vi "Read String.vi"(8 "error in (no error)":errorcluster, 9 "offset (0)":i64, 10 "bytes to read":i64, 11 "pointer in":u64) -> (0 "error out":errorcluster, 1 "offset out":i64, 2 "string out":string, 3 "pointer out":u64)   [LabVIEW 2013, in "Linux RT IPC.Shared Memory.lvlib"]
uses:
  Linux RT IPC.Shared Memory.lvlib
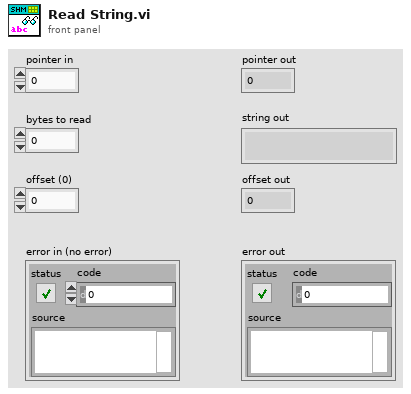
[diagram p1: front panel]
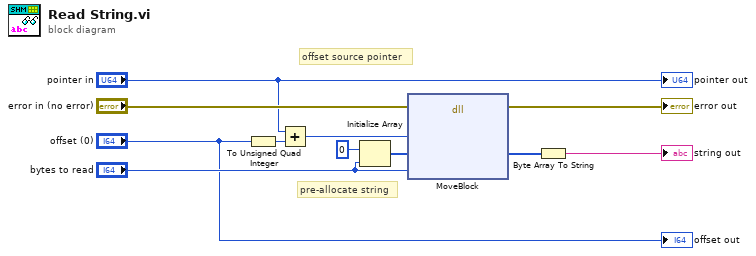
[diagram p0: block diagram]
diagram:
  # "pre-allocate string"
  # "offset source pointer"
  n1 = To Unsigned Quad Integer(1:"offset (0)") -> (0:w6:u64)
  n2 = Add(x="pointer in", y=w6) -> (x+y=w3:u64)
  n3 = Initialize Array(u8 0, "bytes to read") -> (w4:u8[])
  n4 = dll-call lib="LabVIEW" fn="MoveBlock"(error in="error in (no error)", "pointer"=w3, "data"=w4, "size"="bytes to read") -> (error out=→"error out":errorcluster, "data"=w2:u8[])  [unwired: 5 in, 1 out]
  n5 = Byte Array To String(unsigned byte array=w2) -> (string=→"string out":string)
  "pointer out" <- "pointer in"
  "offset out" <- "offset (0)"
